vi "Configure Channel.vi"(8 "error in":errorcluster, 11 "Continuous Waveforn Acq CFG in":refnum<class "Continuous Waveform Acq CFG.lvclass">) -> (0 "error out":errorcluster, 3 "Continuous Waveforn Acq CFG out":refnum<class "Continuous Waveform Acq CFG.lvclass">)   [LabVIEW 2023, in "RIGOL DS1054.lvlib" / "Continuous Waveform Acq CFG.lvclass"]
uses:
  Continuous Waveform Acq CFG.lvclass
  <instrlib>/RIGOL DS1000 Series/RIGOL DS1000 Series.lvlib
  <vilib>/ErrorRing/Error Ring.xnode
  <vilib>/Utility/error.llb/Error Cluster From Error Code.vi
  Scope VISA/Configuration/Scope VISA CFG.lvclass
  Configuration Base/Configuration Base.lvclass
  <vilib>/JDP Science/JSONtext/JSONtext.lvlib
  13379d92-62cc-4363-acda-c88c807c27a1.vi
  9b939277-0290-4c63-9551-43f1276b4dba.vi
  0b58aace-1cbd-4074-a164-6438e127f828.vi
  b8864795-ac20-4438-a1f8-eecbd4742ffa.vi
  e8d34bdc-91e5-4007-9163-e62f6bb2c44f.vi
  cf25363e-02e6-4a10-b51f-04386fb50273.vi
  0f5d0d8d-dd60-44e3-8a05-a79d933c3f09.vi
  D:/git/HAL/Scope VISA/Configuration/Scope VISA CFG.lvclass
  D:/git/HAL/Scope Base/Configuration/Scope Base CFG.lvclass
  D:/git/HAL/Configuration Base/Configuration Base.lvclass
  D:/git/HAL/Interfaces/IConfigure/IConfigure.lvclass
  D:/git/HAL/Devices/Rigol DS1054/Configurations/Acquire Continuous Waveform/Continuous Waveform Acq CFG.lvclass
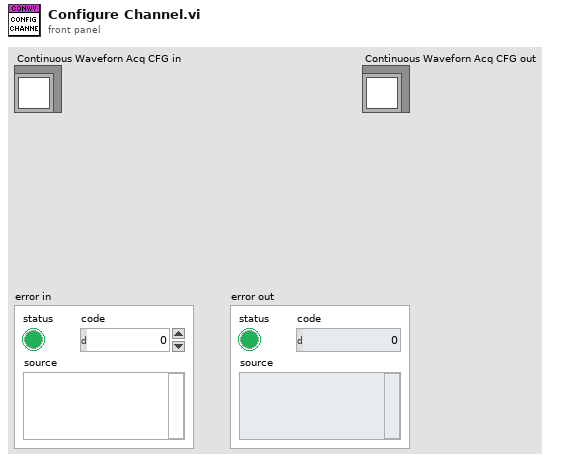
[diagram p1: front panel]
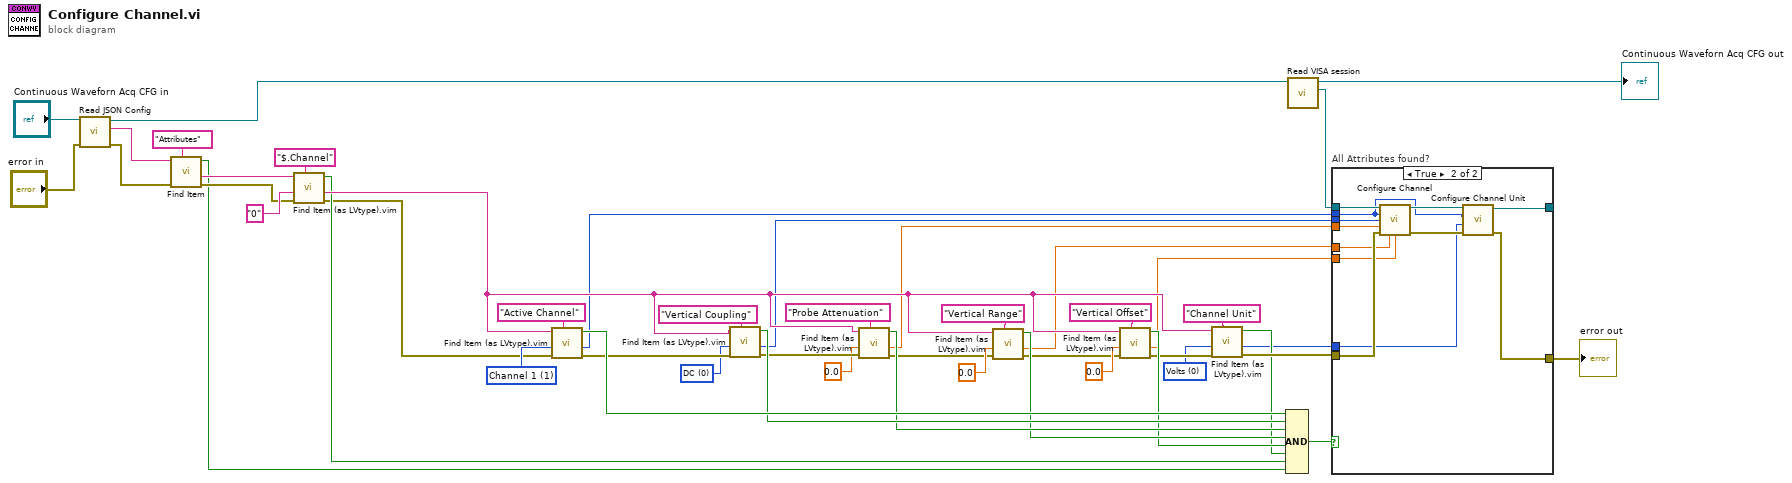
[diagram p0: block diagram]
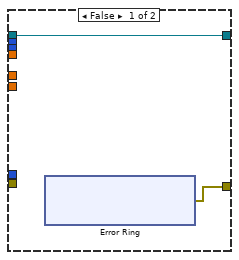
[diagram p2: hidden frame]
diagram:
  w5 = u16 0 items=["DC", "AC", "Ground"] ("Vertical Coupling (0: DC)")
  w6 = u16 1 items=["Channel 1"=1, "Channel 2"=2, "Channel 3"=3, "Channel 4"=4] ("Channel (1: Channel 1)")
  w9 = u16 0 items=["Volts", "Amperes", "Watts", "Unknown"] ("Unit (0: Volts)")
  n1 = call "Read JSON Config.vi"("error in (no error)"="error in", "object in"="Continuous Waveforn Acq CFG in") -> ("error out"=w41:errorcluster, "<JSON>Config"=w44:string, "object out"=w43:refnum<class "Continuous Waveform Acq CFG.lvclass">)  [unwired: 7 in]
  n2 = call <vilib>:"Find Item.vi"("$Path or Item Name"="Attributes", "error in (no error)"=w41, "JSON"=w44) -> ("error out"=w36:errorcluster, "<JSON>"=w39:string, "Found"=w3:bool)  [unwired: 5 in, 1 out]
  n3 = call "Find Item (as LVtype).vim"("$Path or Item Name"="$.Channel", "error in (no error)"=w36, "Data Type and Default Value"="0", "JSON"=w39) -> ("error out"=w1:errorcluster, "Data"=w35:string, "Found"=w2:bool)  [unwired: 4 in, 1 out]
  n4 = call "Find Item (as LVtype).vim"("$Path or Item Name"="Active Channel", "error in (no error)"=w1, "Data Type and Default Value"=w6, "JSON"=w35) -> ("error out"=w32:errorcluster, "Data"=w17:u16, "Found"=w34:bool)  [unwired: 4 in, 1 out]
  n5 = call "Find Item (as LVtype).vim"("$Path or Item Name"="Vertical Coupling", "error in (no error)"=w32, "Data Type and Default Value"=w5, "JSON"=w35) -> ("error out"=w30:errorcluster, "Data"=w16:u16, "Found"=w31:bool)  [unwired: 4 in, 1 out]
  n6 = call "Find Item (as LVtype).vim"("$Path or Item Name"="Probe Attenuation", "error in (no error)"=w30, "Data Type and Default Value"=0.0, "JSON"=w35) -> ("error out"=w25:errorcluster, "Data"=w15:dbl, "Found"=w27:bool)  [unwired: 4 in, 1 out]
  n7 = call "Find Item (as LVtype).vim"("$Path or Item Name"="Vertical Range", "error in (no error)"=w25, "Data Type and Default Value"=0.0, "JSON"=w35) -> ("error out"=w19:errorcluster, "Data"=w14:dbl, "Found"=w21:bool)  [unwired: 4 in, 1 out]
  n8 = call "Find Item (as LVtype).vim"("$Path or Item Name"="Vertical Offset", "error in (no error)"=w19, "Data Type and Default Value"=0.0, "JSON"=w35) -> ("error out"=w11:errorcluster, "Data"=w13:dbl, "Found"=w20:bool)  [unwired: 4 in, 1 out]
  n9 = call "Find Item (as LVtype).vim"("$Path or Item Name"="Channel Unit", "error in (no error)"=w11, "Data Type and Default Value"=w9, "JSON"=w35) -> ("error out"=w10:errorcluster, "Data"=w7:u16, "Found"=w8:bool)  [unwired: 4 in, 1 out]
  n10 = Compound Arithmetic op=AND(w34, w31, w27, w21, w20, w8, w2, w3) -> (w18:bool)
  n11 = call "Read VISA session.vi"("Scope VISA CFG in"=w43) -> ("VISA session"=w46:refnum<visa-resource-name>, "Scope VISA CFG out"=→"Continuous Waveforn Acq CFG out":refnum<class "Continuous Waveform Acq CFG.lvclass">)  [unwired: 8 in, 1 out]
  n12 = case "All Attributes found?" shown="True" w18 {
    tunnel: w46 -> [w49 w67]
    tunnel: w17 -> [_ w58]
    tunnel: w16 -> [_ w57]
    tunnel: w15 -> [_ w56]
    tunnel: w10 -> [_ w66]
    tunnel: w14 -> [_ w65]
    tunnel: w13 -> [_ w64]
    tunnel: [w50 w60] -> w48
    tunnel: [w49 w62] -> _
    tunnel: w7 -> [_ w59]
    frame False {
      n13 = xnode "Error Ring"() -> ("error out"=w50:errorcluster)
    }
    frame True {
      n14 = call <instrlib>:"Configure Channel.vi"("VISA resource name"=w67, "Channel (1: Channel 1)"=w58, "Vertical Coupling (0: DC)"=w57, "Probe Attenuation (1.0)"=w56, "error in (no error)"=w66, "Vertical Range (1.0 V)"=w65, "Vertical Offset (0.0 V)"=w64) -> ("VISA resource name out"=w63:refnum<visa-resource-name>, "error out"=w61:errorcluster)  [unwired: 7 in]
      n15 = call <instrlib>:"Configure Channel Unit.vi"("error in (no error)"=w61, "Unit (0: Volts)"=w59, "Channel Name (0: Channel 1)"=w58, "VISA resource name"=w63) -> ("error out"=w60:errorcluster, "VISA resource name out"=w62:refnum<visa-resource-name>)  [unwired: 6 in]
    }
  }
  "error out" <- w48
